vi "LJUD_eGetSS.vi"(5 "Channel":string, 7 "IOType":string, 8 "error in":errorcluster, 10 "Value Write":dbl format="%.2f", 11 "Handle In":i32) -> (0 "error out":errorcluster, 2 "Value Read":dbl format="%.2f", 3 "Handle Out":i32)   [LabVIEW 2016]
uses:
  labjackud.dll
panel:
  in  "x1":i32
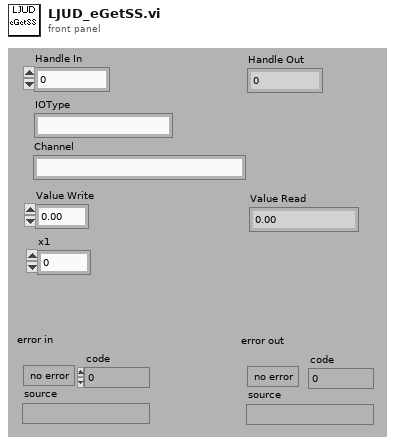
[diagram p1: front panel]
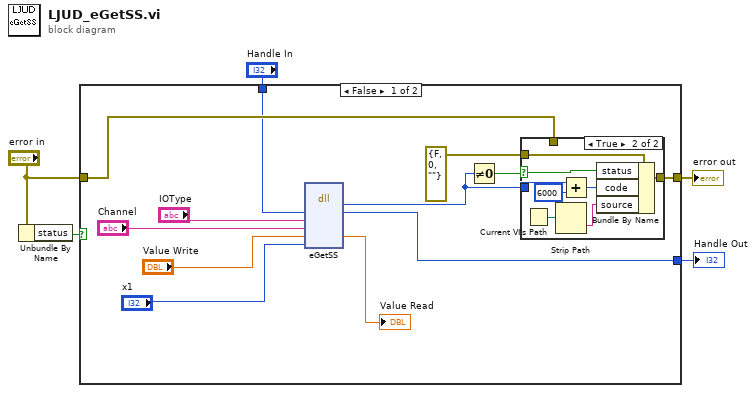
[diagram p0: block diagram]
diagram:
  n1 = Unbundle By Name("error in") -> ("status"=w4:bool)
  n2 = case shown="False" w4 {
    tunnel: [w14 w28] -> w5
    tunnel: "error in" -> [w8 w28]
    tunnel: "Handle In" -> [w7 w27]
    tunnel: [w6 w27] -> w1
    frame False {
      n3 = dll-call lib="labjackud.dll" fn="eGetSS"("Handle"=w7, "IOType"="IOType", "Channel"="Channel", "Value"="Value Write", "x1"="x1") -> (w11:i32, "Handle"=w6:i32, "Value"=→"Value Read":dbl)  [unwired: 6 in, 2 out]
      n4 = Not Equal To 0?(x=w11) -> (x != 0?=w12:bool)
      n5 = case shown="True" w12 {
        selector: w12 -> [_ w25]
        tunnel: [w18 w26] -> w14
        tunnel: errorcluster {"status"=FALSE, "code"=0, "source"=""} ("error IO") -> [_ w24]
        tunnel: w11 -> [_ w20]
        tunnel: w8 -> [w18 _]
        frame False {
        }
        frame True {
          n6 = Current VI's Path() -> (path=w22:path)
          n7 = Strip Path(path=w22) -> (name=w23:string)  [unwired: 1 out]
          n8 = Add(x=w20, y=6000) -> (x+y=w21:i32)
          n9 = Bundle By Name(cluster=w24, "status"=w25, "code"=w21, "source"=w23) -> (w26:errorcluster)
        }
      }
    }
    frame True {
    }
  }
  "error out" <- w5
  "Handle Out" <- w1
